vi "AFT Set Coefficients (FIR, Real).vi"(8 "error in (no error)":errorcluster, 10 "coefficients":dbl[](array[numeric]), 11 "adaptive filter in":refnum<k20>) -> (0 "error out":errorcluster, 3 "adaptive filter out":refnum<k20>)   [LabVIEW 2017, in "NI_AdaptiveFilter.lvlib"]
doc: "Sets the coefficients of an adaptive filter that you create with the least mean squares (LMS) or recursive least squares (RLS) algorithms. You must manually select the polymorphic instance you want to use."
uses:
  <vilib>/addons/Adaptive Filters/NI_AdaptiveFilter.lvlib
  <resource>/AdaptiveFilters.dll
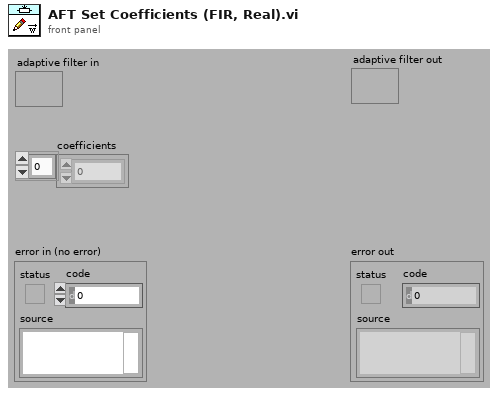
[diagram p1: front panel]
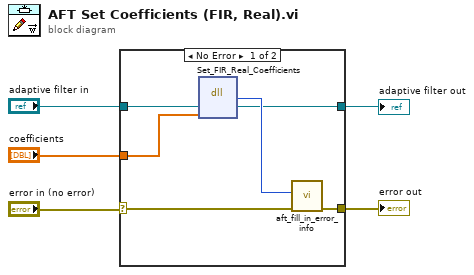
[diagram p0: block diagram]
diagram:
  n1 = case shown="No Error" "error in (no error)" {
    selector: "error in (no error)" -> [w11 w13]
    tunnel: [w9 w13] -> w5
    tunnel: "adaptive filter in" -> [w7 w12]
    tunnel: [w6 w12] -> w1
    tunnel: "coefficients" -> [w8 _]
    frame No Error {
      n2 = dll-call lib="C:/Program Files/National Instruments/LabVIEW 2017/resource/AdaptiveFilters.dll" fn="Set_FIR_Real_Coefficients"("pSession"=w7, "Coefficients"=w8) -> ("err"=w10:i32, "pSession"=w6:refnum<k20>)  [unwired: 4 in, 2 out]
      n3 = call <vilib>:"aft_fill_in_error_info.vi"("error in"=w11, "status code"=w10) -> ("error out"=w9:errorcluster)  [unwired: 2 in, 7 out]
    }
    frame Error {
    }
  }
  "error out" <- w5
  "adaptive filter out" <- w1
